vi "update-image-data-with-new-row.vi"(4 "detrend":bool=TRUE, 6 "data-valid":bool, 9 "iterator":i32, 10 "master-image-data-n":dbl[][](array[numeric]), 11 "avg-data-row":dbl[](array[numeric])) -> (3 "master-image-data-out":dbl[][](array[numeric]))   [LabVIEW 2017]
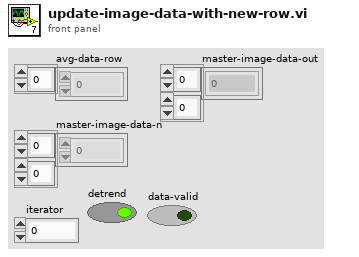
[diagram p1: front panel]
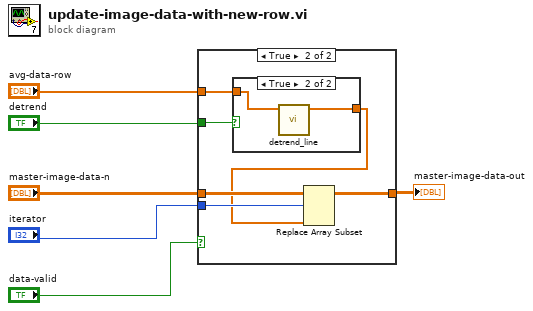
[diagram p0: block diagram]
diagram:
  n1 = case shown="True" "data-valid" {
    tunnel: "iterator" -> [_ w13]
    tunnel: [w7 w12] -> w5
    tunnel: "master-image-data-n" -> [w7 w11]
    tunnel: "detrend" -> [_ w9]
    tunnel: "avg-data-row" -> [_ w8]
    frame False {
    }
    frame True {
      n2 = case shown="True" w9 {
        tunnel: w8 -> [w14 w16]
        tunnel: [w14 w15] -> w10
        frame False {
        }
        frame True {
          n3 = call "detrend_line.vi"("data_in"=w16) -> ("detrended"=w15:dbl[])  [unwired: 10 in]
        }
      }
      n4 = Replace Array Subset(array=w11, new element=w10, index (row)=w13) -> (w12:dbl[][])  [unwired: 1 in]
    }
  }
  "master-image-data-out" <- w5
